vi "Set Sides.vi"(8 "error in (no error)":errorcluster, 10 "Sides":refnum<class "Line.lvclass">[](array[class]), 11 "Polygon.lvclass in":refnum<class "Polygon.lvclass">) -> (0 "error out":errorcluster, 3 "Polygon.lvclass out":refnum<class "Polygon.lvclass">)   [LabVIEW 2020, in "Polygon.lvclass"]
uses:
  Polygon.lvclass
  Line/Line.lvclass
  Polygon.lvclass/Polygon.ctl
panel:
  # "expressionflow.com"
  # "Copyright (c) 2008 Tomi Maila. All rights reserved."
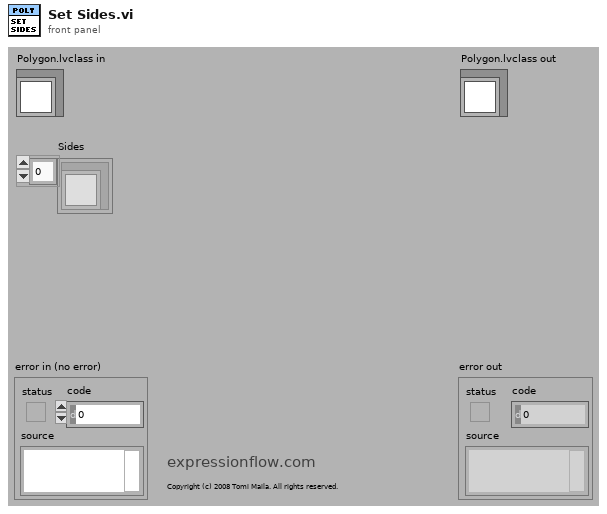
[diagram p1: front panel]
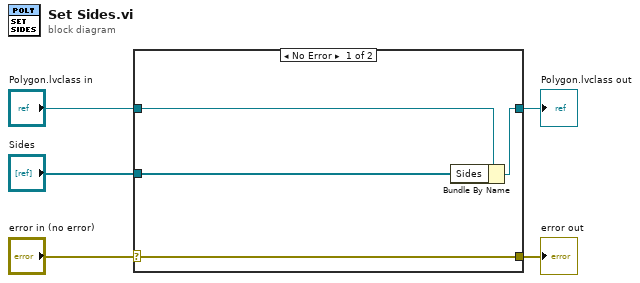
[diagram p0: block diagram]
diagram:
  n1 = case shown="No Error" "error in (no error)" {
    selector: "error in (no error)" -> [w9 w10]
    tunnel: [w9 w10] -> w4
    tunnel: [w7 w11] -> w2
    tunnel: "Polygon.lvclass in" -> [w8 w11]
    tunnel: "Sides" -> [w6 _]
    frame No Error {
      n2 = Bundle By Name(cluster=w8, "Sides"=w6) -> (w7:refnum<class "Polygon.lvclass">)
    }
    frame Error {
    }
  }
  "error out" <- w4
  "Polygon.lvclass out" <- w2
